vi "DoPaint.vi"(8 "error in (no error)":errorcluster, 11 "Paint in":refnum<class "Paint.lvclass">) -> (0 "error out":errorcluster, 3 "Paint out":refnum<class "Paint.lvclass">)   [LabVIEW 2014, in "Paint.lvclass"]
uses:
  Paint.lvclass
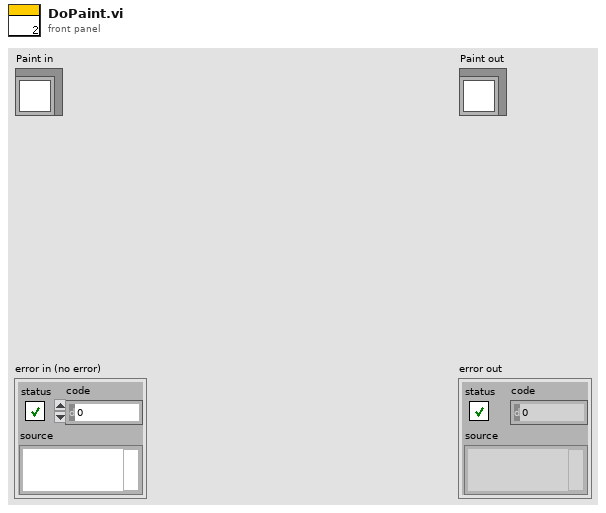
[diagram p1: front panel]
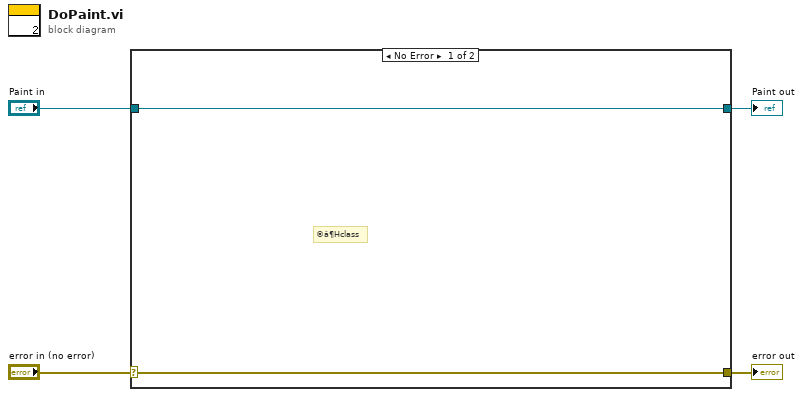
[diagram p0: block diagram]
diagram:
  n1 = case shown="No Error" "error in (no error)" {
    selector: "error in (no error)" -> [w5 w8]
    tunnel: [w5 w8] -> w3
    tunnel: [w6 w7] -> w1
    tunnel: "Paint in" -> [w6 w7]
    frame No Error {
      # "©â¶Hclass"
    }
    frame Error {
    }
  }
  "error out" <- w3
  "Paint out" <- w1
